vi "Bitmap File Writer.vi"(8 "error in":errorcluster, 11 "Color Array":cluster{"Red":u8, "Green":u8, "Blue":u8}[][](array[cluster])) -> (0 "error out":errorcluster)   [LabVIEW 2012, in "paint Xcontrol.xctl"]
uses:
  paint Xcontrol.xctl
  Instance           1 26Saved   Bitmap File Writer .vi
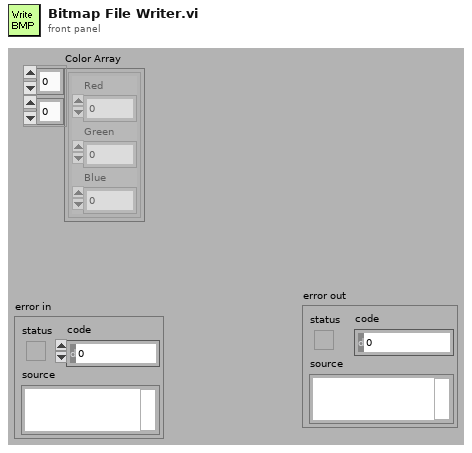
[diagram p1: front panel]
types:
  T1 = enum16{"open", "replace", "create", "open or create", "replace or create", "replace or create with confirmation"}
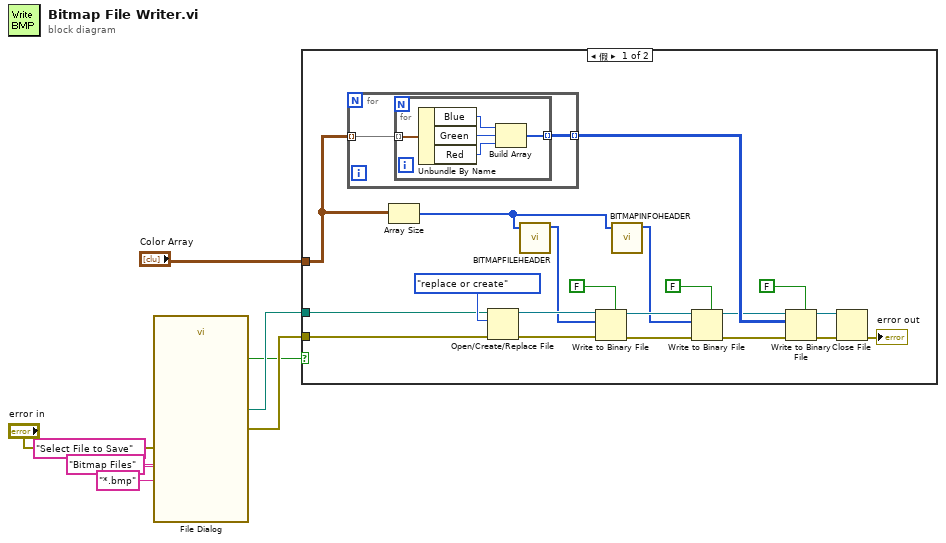
[diagram p0: block diagram]
diagram:
  n1 = call "File Dialog"("prompt"="Select File to Save", "error in"="error in", "pattern (all files)"="*.bmp", "pattern label"="Bitmap Files") -> ("selected path"=w8:path, "cancelled"=w1:bool, "error out"=w7:errorcluster)  [unwired: 8 in, 1 out]
  n2 = case shown="假" w1 {
    tunnel: w8 -> [w12 _]
    tunnel: w7 -> [w11 _]
    tunnel: "Color Array" -> [w10 _]
    frame False {
      n3 = for {
        tunnel: w10 -> [w30] mode=indexing
        tunnel: [w29] -> w17 mode=indexing
        n4 = for {
          tunnel: w30 -> [w35] mode=indexing
          tunnel: [w31] -> w29 mode=indexing
          n5 = Unbundle By Name(w35) -> ("Blue"=w33:u8, "Green"=w34:u8, "Red"=w32:u8)
          n6 = Build Array(w33, w34, w32) -> (w31:u8[])
        }
      }
      n7 = Array Size(array=w10) -> (size(s)=w21:i32[])
      n8 = Open/Create/Replace File(file path (use dialog)=w12, error in=w11, operation (0:open)=T1."replace or create") -> (refnum out=w25:refnum<file>, error out=w24:errorcluster)  [unwired: 3 in, 1 out]
      n9 = call "BITMAPFILEHEADER.vi"("Image Dimensions"=w21) -> ("BITMAPFILEHEADER"=w20:u8[])  [unwired: 10 in]
      n10 = Write to Binary File(file (use dialog)=w25, data=w20, error in=w24, 5:FALSE ("prepend array or string size? (T)")) -> (refnum out=w23:refnum<file>, error out=w22:errorcluster)  [unwired: 2 in, 1 out]
      n11 = call "BITMAPINFOHEADER.vi"("Image Dimensions"=w21) -> ("BITMAPFILEHEADER"=w19:u8[])  [unwired: 10 in]
      n12 = Write to Binary File(file (use dialog)=w23, data=w19, error in=w22, 5:FALSE ("prepend array or string size? (T)")) -> (refnum out=w16:refnum<file>, error out=w15:errorcluster)  [unwired: 2 in, 1 out]
      n13 = Write to Binary File(file (use dialog)=w16, data=w17, error in=w15, 5:FALSE ("prepend array or string size? (T)")) -> (refnum out=w13:refnum<file>, error out=w14:errorcluster)  [unwired: 2 in, 1 out]
      n14 = Close File(refnum=w13, error in=w14) -> (error out=→"error out":errorcluster)  [unwired: 1 out]
    }
    frame True {
    }
  }
